vi "AlliGator [Z] to Z Plot.vi"(8 "Error In":errorcluster, 9 "Phasor Graph Slide (-1: last)":i32=-1, 10 "Single Point Display? (F)":bool, 11 "[Calibrated Phasor]":T1[](array[typedef])) -> (0 "Error Out":errorcluster, 3 "Calibrated Phasor Plot":cluster{"Array":dbl[], "Array":dbl[]})   [LabVIEW 2021, in "AlliGator Phasor Calibration.lvlib"]
doc: "Returns full plot of the series of phasors, or only one if <B>Single Point Display</B> = True.\n\nThe <B>Phasor Graph Slide</B> sepecifies which point to display."
uses:
  AlliGator Phasor Calibration.lvlib
  Phasor/Phasor (g, s).ctl
  ac0ce6f8-85b7-41c8-85c3-d4d04f84f1e4.vi
  18744cc5-2d74-4d38-ba8f-23fcda318c75.vi
  Arrays/Signed Array Index.vi
  Phasor/Phasor.lvlib
panel:
  # "see the AlliGator License on the block diagram (Ctrl+E or Window:Show Block Diagram)"
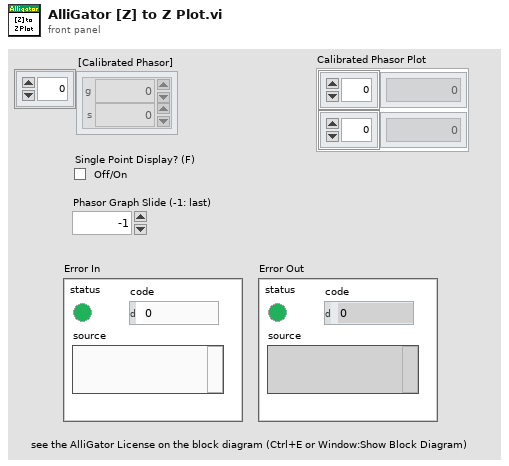
[diagram p1: front panel]
types:
  T1 = typedef "Phasor.lvlib/Phasor (g, s).ctl" = cluster{"g":dbl, "s":dbl}
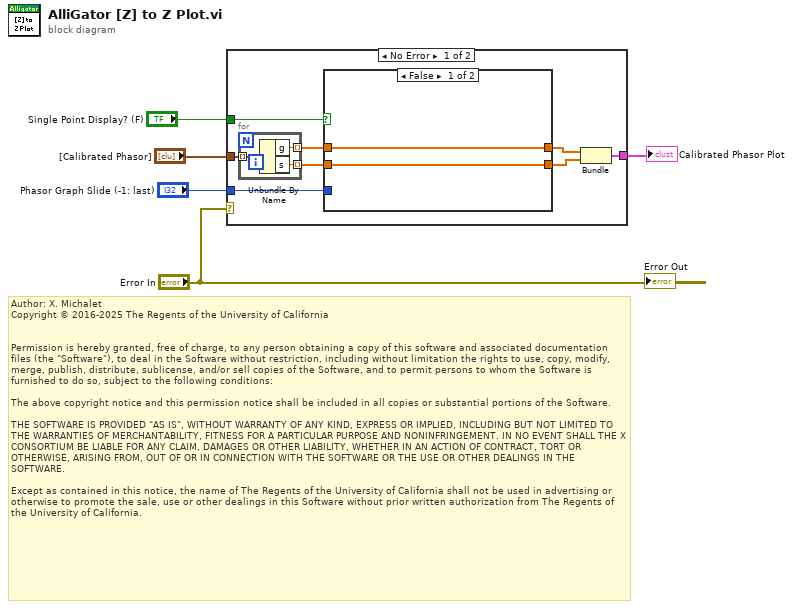
[diagram p0: block diagram]
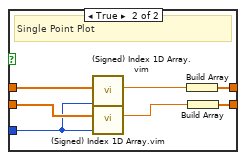
[diagram p2: hidden frame]
diagram:
  # "Author: X. Michalet\nCopyright © 2016-2025 The Regents of the University of California\n \n\nPermission is hereby granted, free of charge, to any person obtaining a copy of this software and associated documentation files (the \"Software\"), to deal in the Software without restriction, including without limitation the rights to use, copy, modify, merge, publish, distribute, sublicense, and/or sell copies of the Software, and to permit persons to whom the Software is furnished to do so, subject to the following conditions:\n\nThe above copyright notice and this permission notice shall be included in all copies or substantial portions of the Software.\n\nTHE SOFTWARE IS PROVIDED \"AS IS\", WITHOUT WARRANTY OF ANY KIND, EXPRESS OR IMPLIED, INCLUDING BUT NOT LIMITED TO THE WARRANTIES OF MERCHANTABILITY, FITNESS FOR A PARTICULAR PURPOSE AND NONINFRINGEMENT. IN NO EVENT SHALL THE X CONSORTIUM BE LIABLE FOR ANY CLAIM, DAMAGES OR OTHER LIABILITY, WHETHER IN AN ACTION OF CONTRACT, TORT OR OTHERWISE, ARISING FROM, OUT OF OR IN CONNECTION WITH THE SOFTWARE OR THE USE OR OTHER DEALINGS IN THE SOFTWARE.\n\nExcept as contained in this notice, the name of The Regents of the University of California shall not be used in advertising or otherwise to promote the sale, use or other dealings in this Software without prior written authorization from The Regents of the University of California."
  n1 = case shown="No Error" "Error In" {
    tunnel: [w13 _] -> w5
    tunnel: "Phasor Graph Slide (-1: last)" -> [w10 _]
    tunnel: "Single Point Display? (F)" -> [w9 _]
    tunnel: "[Calibrated Phasor]" -> [w8 _]
    frame No Error {
      n2 = for {
        tunnel: w8 -> [w25] mode=indexing
        tunnel: [w24] -> w7 mode=indexing
        tunnel: [w23] -> w6 mode=indexing
        n3 = Unbundle By Name(w25) -> ("g"=w24:dbl, "s"=w23:dbl)
      }
      n4 = case shown="False" w9 {
        tunnel: w10 -> [_ w20]
        tunnel: [w15 w17] -> w11
        tunnel: [w14 w16] -> w12
        tunnel: w7 -> [w15 w22]
        tunnel: w6 -> [w14 w21]
        frame False {
        }
        frame True {
          # "Single Point Plot"
          n5 = call "(Signed) Index 1D Array.vim"("Signed Index"=w20, "Array"=w22) -> ("Array Element"=w19:dbl)  [unwired: 9 in]
          n6 = call "(Signed) Index 1D Array.vim"("Signed Index"=w20, "Array"=w21) -> ("Array Element"=w18:dbl)  [unwired: 9 in]
          n7 = Build Array(w19) -> (w17:dbl[])
          n8 = Build Array(w18) -> (w16:dbl[])
        }
      }
      n9 = Bundle(w11, w12) -> (w13:cluster{dbl[], dbl[]})  [unwired: 1 in]
    }
    frame Error {
    }
  }
  "Calibrated Phasor Plot" <- w5
  "Error Out" <- "Error In"
